vi "OAT Torsional Vibration (Analog Tacho) (Waveform) (1 Ch).vi"(0 "analog tacho signal":waveform(dbl)={"t0"=timestamp(0 s since 1904-01-01), "dt"=0.0, "Y"=[]}, 1 "threshold (auto)":dbl=inf format="%.2f", 2 "pulse/revolution (1)":i32=1 min=1, 3 "hysteresis (0)":dbl format="%.2f", 4 "torsional vibration units":enum16{"RPM", "deg/s", "rad/s"}(ring), 5 "error in (no error)":errorcluster, 6 "missing pulses? (no:F)":bool, 7 "pulse width (2)":i32=2 min=0, 8 "reset? (F)":bool, 9 "slope (Rising)":u16(ring) items=["Rising", "Falling"], 10 "compensate geometric imperfection? (F)":bool, 11 "output interval [s]":dbl=0.001 min=0.0) -> (14 "torsional vibration signal":waveform(dbl), 15 "speed profile":T1 {"speed [RPM]" format="%.2f"; "time [s]" format="%.2f"}, 18 "unit label":string, 19 "error out":errorcluster)   [LabVIEW 2017, in "SoundVib_Torsional.lvlib"]
doc: "Calculates torsional vibration signals from analog tachometer signals. This VI can return torsional vibration signals as either waveform signals or even-angle signals. Wire data to the <B>analog tacho signal</B> input to determine the polymorphic instance to use or manually select the instance."
uses:
  <vilib>/addons/Sound and Vibration/Order Analysis/Torsional Vibration/SoundVib_Torsional.lvlib
  <vilib>/addons/Sound and Vibration/Order Analysis/Tach Process/SubVIs/speed profile.ctl
  <vilib>/addons/_NISVFA/_Shared subVIs/Common/svc_Check for Waveform Parameter Continuity (no state).vi
  <vilib>/addons/_NISVFA/_Shared subVIs/Common/svc_Get SV Channel Info.vi
  <vilib>/addons/_NISVFA/_Shared subVIs/Common/svc_Engineering Units to Unit Label.vi
  <vilib>/addons/_NISVFA/_Shared subVIs/Common/svc_Unit Label to Engineering Units.vi
  <vilib>/addons/Sound and Vibration/Order Analysis/Tach Process/SoundVib_TachProcess.lvlib
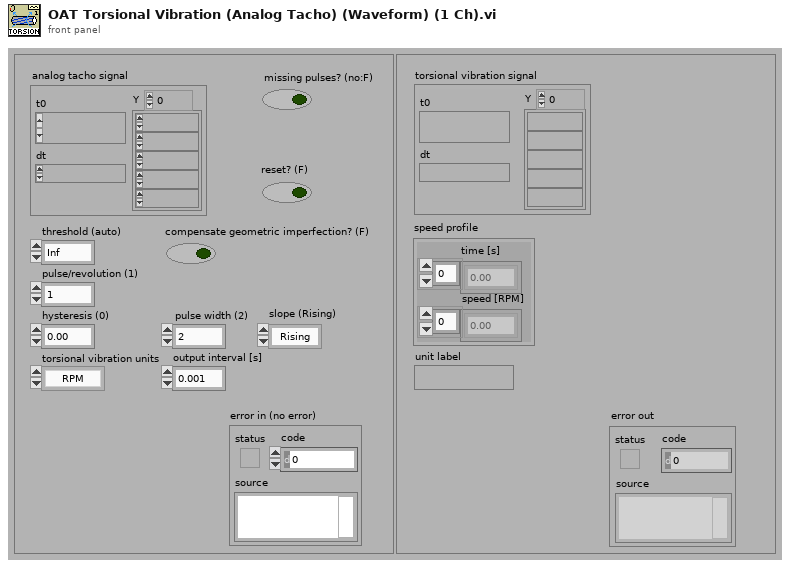
[diagram p1: front panel]
types:
  T1 = typedef "SoundVib_TachProcess.lvlib/speed profile.ctl" = cluster{"time [s]":dbl[], "speed [RPM]":dbl[]}
  T2 = cluster{"dt":bool, "t0 continuity":bool, "array length":bool, "channel info":bool, "name":bool}
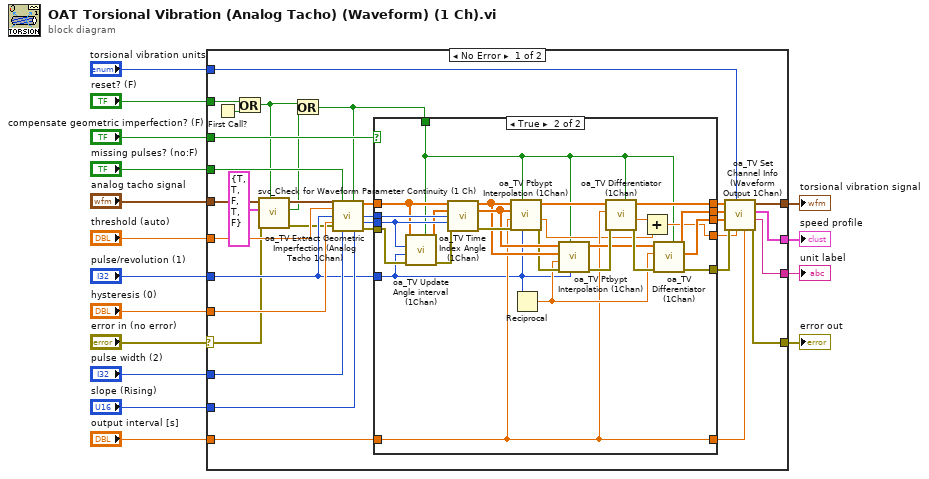
[diagram p0: block diagram]
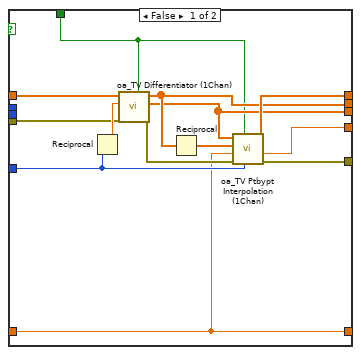
[diagram p2: hidden frame]
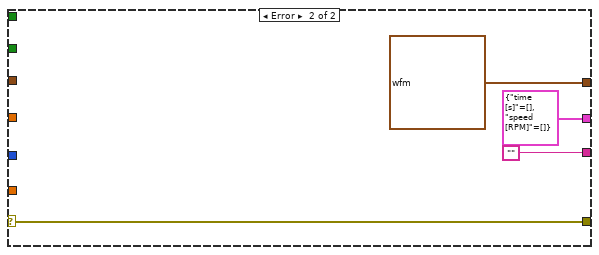
[diagram p3: hidden frame]
diagram:
  n1 = case shown="No Error" "error in (no error)" {
    selector: "error in (no error)" -> [w22 w91]
    tunnel: "analog tacho signal" -> [w49 _]
    tunnel: "threshold (auto)" -> [w48 _]
    tunnel: "pulse/revolution (1)" -> [w39 _]
    tunnel: "pulse width (2)" -> [w47 _]
    tunnel: "slope (Rising)" -> [w46 _]
    tunnel: "hysteresis (0)" -> [w45 _]
    tunnel: [w34 waveform(dbl) {"t0"=timestamp(0 s since 1904-01-01), "dt"=1.0, "Y"=[]} ("even time speed")] -> w11
    tunnel: [w33 w91] -> w10
    tunnel: "compensate geometric imperfection? (F)" -> [w27 _]
    tunnel: "reset? (F)" -> [w42 _]
    tunnel: "output interval [s]" -> [w31 _]
    tunnel: "torsional vibration units" -> [w32 _]
    tunnel: [w29 T1 {"time [s]"=[], "speed [RPM]"=[]} ("speed profile")] -> w3
    tunnel: [w25 ""] -> w2
    tunnel: "missing pulses? (no:F)" -> [w24 _]
    frame No Error {
      n2 = First Call?() -> (First Call?: T/F=w43:bool)
      n3 = Or(x=w42, y=w43) -> (x .or. y?=w19:bool)
      n4 = call <vilib>:"svc_Check for Waveform Parameter Continuity (1 Ch).vi"("restart averaging (F)"=w19, "error in (no error)"=w22, "checks for channel parameter change"=T2 {"dt"=TRUE, "t0 continuity"=TRUE, "array length"=FALSE, "channel info"=TRUE, "name"=FALSE}, "scaled signal [EU]"=w49) -> ("error out"=w21:errorcluster, "waveform parameter changed"=w18:bool, "dup scaled signal [EU]"=w23:waveform(dbl))  [unwired: 2 in, 3 out]
      n5 = Or(x=w19, y=w18) -> (x .or. y?=w20:bool)
      n6 = call <vilib>:"oa_TV Extract Geometric Imperfection (Analog Tacho 1Chan).vi"("analog tacho signal"=w23, "missing pulses? (no:F)"=w24, "reset? (F)"=w20, "threshold (auto)"=w48, "pulse/revolution"=w39, "hysteresis(0)"=w45, "error in (no error)"=w21, "pulse width (2)"=w47, "slope (Rising)"=w46) -> ("pulse positions"=w40:dbl[], "revulotion"=w41:i32, "revulotion index"=w38:i32, "error out"=w44:errorcluster)  [unwired: 3 in]
      n7 = case shown="True" w27 {
        tunnel: w44 -> [w60 w69]
        tunnel: w41 -> [_ w70]
        tunnel: w40 -> [w62 w66]
        tunnel: w39 -> [w59 w68]
        tunnel: w38 -> [_ w67]
        tunnel: [w52 w80] -> w37
        tunnel: [w57 w79] -> w36
        tunnel: [w55 w78] -> w35
        tunnel: w31 -> [w51 w74]
        tunnel: [w53 w71] -> w30
        tunnel: [w54 w75] -> w28
        tunnel: [w51 w74] -> w26
        tunnel: w20 -> [w50 w63]
        frame False {
          n8 = Reciprocal(x=w59) -> (1/x=w61:dbl)
          n9 = call <vilib>:"oa_TV Differentiator (1Chan).vi"("reset? (True)"=w50, "error in (no error)"=w60, "deltaX"=w61, "Y[n]"=w62) -> ("error out"=w58:errorcluster, "X[n]"=w54:dbl[], "dY[n]/dX[n]"=w55:dbl[])  [unwired: 4 in, 1 out]
          n10 = Reciprocal(x=w55) -> (1/x=w56:dbl[])
          n11 = call <vilib>:"oa_TV Ptbypt Interpolation (1Chan).vi"("buffer size"=w59, "reset? (F)"=w50, "error in (no error)"=w58, "dX"=w51, "Y"=w56, "X"=w54) -> ("error out"=w52:errorcluster, "X0"=w53:dbl, "resampled Y"=w57:dbl[])  [unwired: 2 in, 1 out]
        }
        frame True {
          n12 = call <vilib>:"oa_TV Update Angle interval (1Chan).vi"("reset? (F)"=w63, "error in (no error)"=w69, "pulse/revolution"=w68, "revulotion index"=w67, "pulse positions"=w66) -> ("error out"=w64:errorcluster, "angle intervals"=w65:dbl[])  [unwired: 5 in]
          n13 = call <vilib>:"oa_TV Time Index Angle (1Chan).vi"("pulse positions"=w66, "angle intervals"=w65, "revolution"=w70, "revolution index"=w67, "error in (no error)"=w64) -> ("pulse positions"=w85:dbl[], "angle"=w86:dbl[], "error out"=w87:errorcluster)  [unwired: 8 in]
          n14 = call <vilib>:"oa_TV Ptbypt Interpolation (1Chan).vi"("buffer size"=w68, "reset? (F)"=w63, "error in (no error)"=w87, "dX"=w74, "Y"=w86, "X"=w85) -> ("error out"=w84:errorcluster, "X0"=w72:dbl, "resampled Y"=w83:dbl[])  [unwired: 2 in, 1 out]
          n15 = Reciprocal(x=w68) -> (1/x=w77:dbl)
          n16 = call <vilib>:"oa_TV Ptbypt Interpolation (1Chan).vi"("buffer size"=w68, "reset? (F)"=w63, "error in (no error)"=w84, "dX"=w77, "Y"=w85, "X"=w86) -> ("error out"=w82:errorcluster, "resampled Y"=w76:dbl[])  [unwired: 2 in, 2 out]
          n17 = call <vilib>:"oa_TV Differentiator (1Chan).vi"("reset? (True)"=w63, "error in (no error)"=w82, "deltaX"=w74, "Y[n]"=w83) -> ("error out"=w81:errorcluster, "Delay"=w73:dbl, "dY[n]/dX[n]"=w79:dbl[])  [unwired: 4 in, 1 out]
          n18 = Add(x=w73, y=w72) -> (x+y=w71:dbl)
          n19 = call <vilib>:"oa_TV Differentiator (1Chan).vi"("reset? (True)"=w63, "error in (no error)"=w81, "deltaX"=w77, "Y[n]"=w76) -> ("error out"=w80:errorcluster, "X[n]"=w75:dbl[], "dY[n]/dX[n]"=w78:dbl[])  [unwired: 4 in, 1 out]
        }
      }
      n20 = call <vilib>:"oa_TV Set Channel Info (Waveform Output 1Chan).vi"("output interval [s]"=w26, "t0"=w30, "torisional vibration unit (RPM)"=w32, "error in (no error)"=w37, "pulse position"=w28, "seconds/rev"=w35, "revolutions/sec"=w36) -> ("error out"=w33:errorcluster, "unit label"=w25:string, "speed profile"=w29:T1, "torsional vibration"=w34:waveform(dbl))  [unwired: 1 in]
    }
    frame Error {
    }
  }
  "torsional vibration signal" <- w11
  "error out" <- w10
  "speed profile" <- w3
  "unit label" <- w2
